vi "Parse Digital Module.vi"(11 "DigitalModule":T1) -> (0 "GPIO Output Enable":bool[](array[boolean]), 1 "GPIO State":bool[](array[boolean]), 2 "PWM":cluster{u8, u8}[](array[slide])=[{128, 128}, {128, 128}, {128, 128}, {128, 128}, {128, 128}, {128, 128}, {128, 128}, {128, 128}, {128, 128}, {128, 128}] scale=1.0..255.0, 3 "Relay":cluster{"Forward":bool[], "Reverse":bool[]})   [LabVIEW 2020]
uses:
  <vilib>/Rock Robotics/WPI/DriverStation/WPI_DriverStationDigitalData.ctl
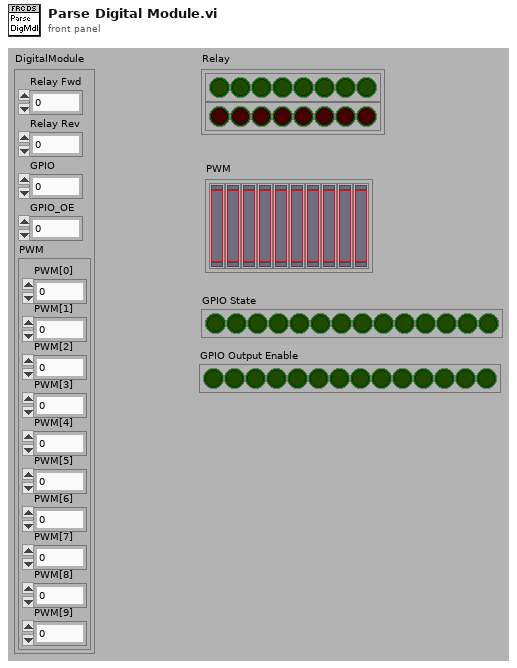
[diagram p1: front panel]
types:
  T1 = typedef "WPI_DriverStationDigitalData.ctl" = cluster{"Relay Fwd":u8, "Relay Rev":u8, "GPIO":u16, "GPIO_OE":u16, "PWM":cluster{"PWM[0]":u8, "PWM[1]":u8, "PWM[2]":u8, "PWM[3]":u8, "PWM[4]":u8, "PWM[5]":u8, "PWM[6]":u8, "PWM[7]":u8, "PWM[8]":u8, "PWM[9]":u8}}
  T2 = cluster{"PWM[0]":u8, "PWM[1]":u8, "PWM[2]":u8, "PWM[3]":u8, "PWM[4]":u8, "PWM[5]":u8, "PWM[6]":u8, "PWM[7]":u8, "PWM[8]":u8, "PWM[9]":u8}
  T3 = cluster{"Boolean array":bool[], "Boolean array":bool[]}
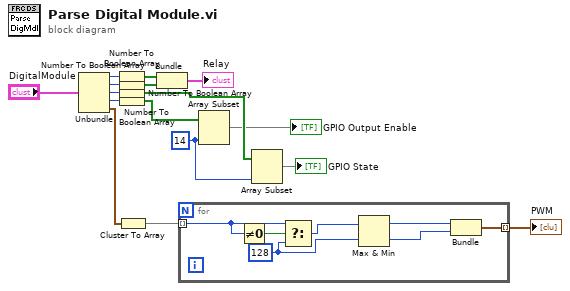
[diagram p0: block diagram]
diagram:
  w4 = 14 ("length")
  n1 = Unbundle("DigitalModule") -> ("Relay Fwd"=w15:u8, "Relay Rev"=w14:u8, "GPIO"=w6:u16, "GPIO_OE"=w7:u16, "PWM"=w13:T2)
  n2 = Number To Boolean Array(number=w15) -> (Boolean array=w12:bool[])
  n3 = Number To Boolean Array(number=w14) -> (Boolean array=w11:bool[])
  n4 = Number To Boolean Array(number=w6) -> (Boolean array=w3:bool[])
  n5 = Number To Boolean Array(number=w7) -> (Boolean array=w5:bool[])
  n6 = Cluster To Array(cluster=w13) -> (array=w9:u8[])
  n7 = Bundle("Boolean array"=w12, "Boolean array"=w11) -> (→"Relay":T3)  [unwired: 1 out]
  n8 = for {
    tunnel: w9 -> [w19] mode=indexing
    tunnel: [w21] -> w8 mode=indexing
    w17 = u8 128 ("f")
    n9 = Not Equal To 0?(x=w19) -> (x != 0?=w20:bool)
    n10 = Select(t=w19, s=w20, f=w17) -> (s? t:f=w18:u8)
    n11 = Max & Min(x=w18, y=w17) -> (max(x,y)=w22:u8, min(x,y)=w23:u8)
    n12 = Bundle(w22, w23) -> (w21:cluster{u8, u8})  [unwired: 1 out]
  }
  "PWM" <- w8
  n13 = Array Subset(array=w5, length=w4) -> (→"GPIO Output Enable":bool[])  [unwired: 1 in]
  n14 = Array Subset(array=w3, length=w4) -> (→"GPIO State":bool[])  [unwired: 1 in]
